vi "Write DetailedResult.vi"(8 "error in (no error)":errorcluster, 10 "DetailedResult":T1, 11 "TestBench in":refnum<class "TestBench.lvclass">) -> (0 "error out":errorcluster, 3 "TestBench out":refnum<class "TestBench.lvclass">)   [LabVIEW 2019, in "TestBench.lvlib" / "TestBench.lvclass"]
uses:
  TestBench.lvclass
  TestBench.lvclass/TestBench.ctl
  LocalReport/LocalReport Messages/Write DetailedResult Msg/Write DetailedResult Msg.lvclass/Write DetailedResult Msg.ctl
  <vilib>/ActorFramework/Message Enqueuer/Message Enqueuer.lvclass/Message Enqueuer.ctl
  <vilib>/ActorFramework/Message Enqueuer/Enqueue.vi
  LocalReport/LocalReport Messages/Write DetailedResult Msg/Write DetailedResult Msg.lvclass
  C:/Program Files (x86)/National Instruments/LabVIEW 2019/vi.lib/ActorFramework/Message/Message.lvclass
  <vilib>/ActorFramework/Message Priority Queue/Priority Enqueue.vi
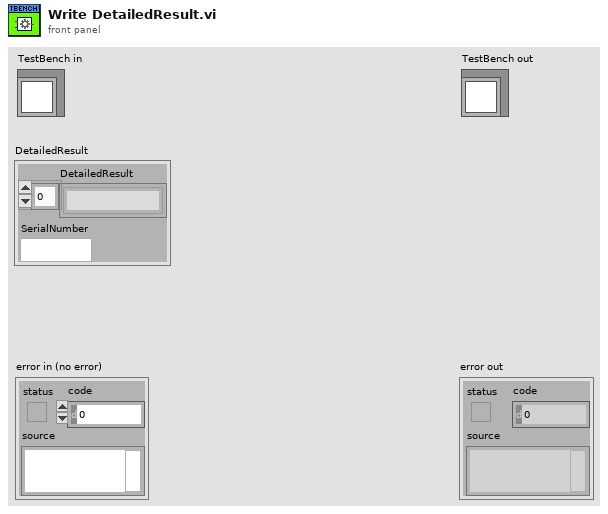
[diagram p1: front panel]
types:
  T1 = cluster{"DetailedResult":string[], "SerialNumber":string}
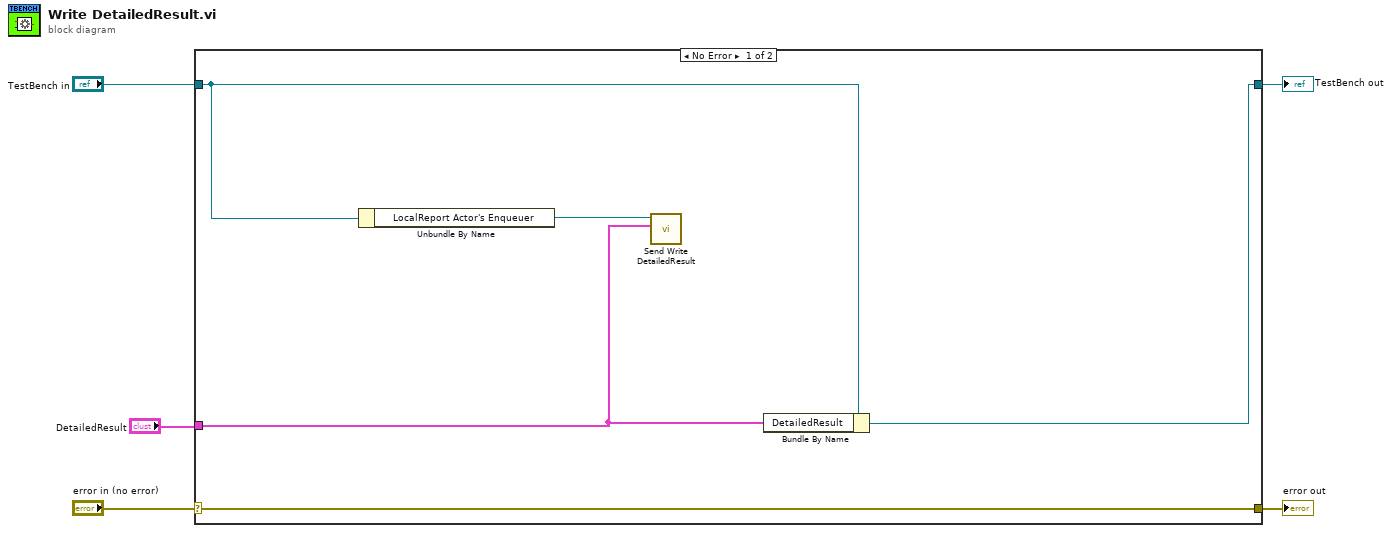
[diagram p0: block diagram]
diagram:
  n1 = case shown="No Error" "error in (no error)" {
    selector: "error in (no error)" -> [w10 w11]
    tunnel: [w10 w11] -> w4
    tunnel: [w9 w12] -> w2
    tunnel: "TestBench in" -> [w8 w12]
    tunnel: "DetailedResult" -> [w6 _]
    frame No Error {
      n2 = Unbundle By Name(w8) -> ("LocalReport Actor's Enqueuer"=w7:refnum<class "Message Enqueuer.lvclass">)
      n3 = call "Send Write DetailedResult.vi"("DetailedResult"=w6, "Message Enqueuer"=w7) -> ()  [unwired: 8 in, 2 out]
      n4 = Bundle By Name(cluster=w8, "DetailedResult"=w6) -> (w9:refnum<class "TestBench.lvclass">)
    }
    frame Error {
    }
  }
  "error out" <- w4
  "TestBench out" <- w2
